vi "ma_sml_Parameter Setting for Zoom Factor.vi"(0 "zoom settings":T1={"zoom"=0, "aliasing protection"=enum."84 dB", "alias protect in transition band"=FALSE, "oversampling ratio"=1.0} {"oversampling ratio" format="%.2f"; "zoom" min=0}, 1 "Reset":bool) -> (2 "CIC Stages":i32, 3 "comb filter order":i32, 4 "interpolation":i32, 5 "filter length":i32, 6 "CFIR par":cluster{"h":dbl[], "M":i32, "N":i32} {"h" format="%.2f"}, 7 "LFIR par":cluster{"h":dbl[], "M":i32, "N":i32} {"h" format="%.2f"})   [LabVIEW 2020, in "NI_MAPro.lvlib"]
uses:
  NI_MAPro.lvlib
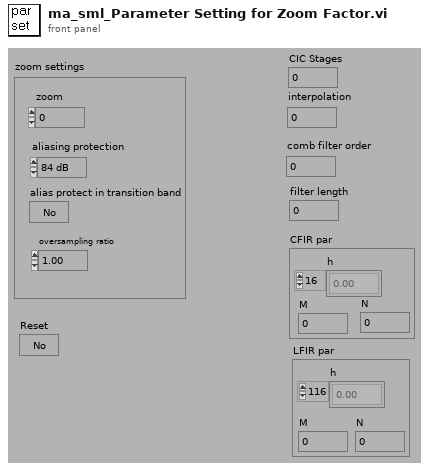
[diagram p1: front panel]
types:
  T1 = cluster{"zoom":i32, "aliasing protection":enum16{"84 dB", "96 dB", "120 dB"}, "alias protect in transition band":bool, "oversampling ratio":dbl}
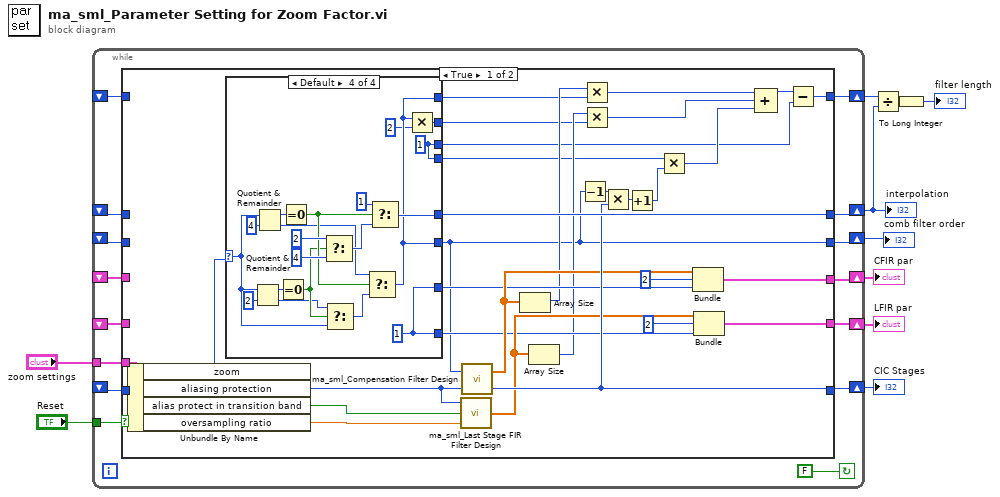
[diagram p0: block diagram]
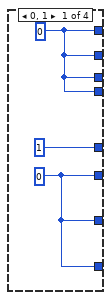
[diagram p2: hidden frame]
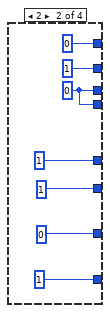
[diagram p3: hidden frame]
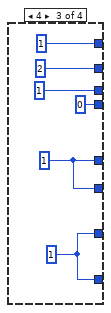
[diagram p4: hidden frame]
diagram:
  n1 = while {
    tunnel: "zoom settings" -> [w11]
    shift-left: _ -> [w14]
    shift-right: [w15] -> w4
    shift-left: _ -> [w16]
    shift-right: [w13] -> w6
    tunnel: "Reset" -> [w17]
    shift-left: _ -> [w18]
    shift-right: [w21] -> w9
    shift-left: _ -> [w19]
    shift-right: [w20] -> w3
    shift-left: _ -> [w22]
    shift-right: [w24] -> w7
    shift-left: _ -> [w23]
    shift-right: [w25] -> w8
    stop <- FALSE continue-if-true
    n2 = case shown="True" w17 {
      tunnel: [w53 w97] -> w25
      tunnel: [w52 w96] -> w24
      tunnel: w23 -> [_ w97]
      tunnel: w22 -> [_ w96]
      tunnel: [w27 w94] -> w21
      tunnel: [w50 w95] -> w20
      tunnel: w19 -> [_ w95]
      tunnel: w18 -> [_ w94]
      tunnel: [w49 w93] -> w13
      tunnel: w16 -> [_ w93]
      tunnel: [w32 w92] -> w15
      tunnel: w14 -> [_ w92]
      tunnel: w11 -> [w43 _]
      frame True {
        n3 = Unbundle By Name(w43) -> ("zoom"=w44:i32, "aliasing protection"=w51:enum16{"84 dB", "96 dB", "120 dB"}, "alias protect in transition band"=w47:bool, "oversampling ratio"=w46:dbl)
        n4 = case shown="Default" w44 {
          selector: w44 -> [_ _ _ w76]
          tunnel: [1 1 w70 w86] -> w50
          tunnel: [w58 1 w70 w74] -> w27
          tunnel: [w58 0 w71 w89] -> w42
          tunnel: [w58 1 w71 w89] -> w36
          tunnel: [w56 0 1 w74] -> w31
          tunnel: [w56 1 2 w75] -> w30
          tunnel: [w56 w59 1 w72] -> w29
          tunnel: [w56 w59 0 w72] -> w26
          frame 0, 1 {
            w56 = 0
            w58 = 0
          }
          frame 2 {
            w59 = 0
          }
          frame 4 {
            w71 = 1
            w70 = 1
          }
          frame Default {
            w72 = 1
            w89 = 1
            n5 = Quotient & Remainder(x=w76, y=2) -> (x-y*floor(x/y)=w88:i32, floor(x/y)=w77:i32)
            n6 = Quotient & Remainder(x=w76, y=4) -> (x-y*floor(x/y)=w90:i32, floor(x/y)=w78:i32)
            n7 = Equal To 0?(x=w88) -> (x = 0?=w79:bool)
            n8 = Equal To 0?(x=w90) -> (x = 0?=w81:bool)
            n9 = Select(t=2, s=w79, f=4) -> (s? t:f=w82:i32)
            n10 = Select(t=w77, s=w79, f=w76) -> (s? t:f=w80:i32)
            n11 = Select(t=w78, s=w81, f=w80) -> (s? t:f=w74:i32)
            n12 = Select(t=1, s=w81, f=w82) -> (s? t:f=w86:i32)
            n13 = Multiply(x=w74, y=2) -> (x*y=w75:i32)
          }
        }
        n14 = call "ma_sml_Last Stage FIR Filter Design.vi"("oversampling rate"=w46, "alias protect in final transition"=w47, "stop band attenuation"=w51) -> ("h"=w45:dbl[])
        n15 = call "ma_sml_Compensation Filter Design.vi"("stop band attenuation"=w51, "M"=w27) -> ("CIC stages"=w49:i32, "filter coefficients"=w48:dbl[])
        n16 = Array Size(array=w48) -> (size(s)=w34:i32)
        n17 = Array Size(array=w45) -> (size(s)=w35:i32)
        n18 = Decrement(x=w27) -> (x-1=w41:i32)
        n19 = Multiply(x=w34, y=w31) -> (x*y=w33:i32)
        n20 = Multiply(x=w35, y=w30) -> (x*y=w28:i32)
        n21 = Multiply(x=w41, y=w49) -> (x*y=w40:i32)
        n22 = Increment(x=w40) -> (x+1=w39:i32)
        n23 = Multiply(x=w26, y=w39) -> (x*y=w38:i32)
        n24 = Bundle("filter coefficients"=w48, 2, w42) -> (w53:cluster{"filter coefficients":dbl[], i32, i32})  [unwired: 1 out]
        n25 = Bundle("h"=w45, 2, w36) -> (w52:cluster{"h":dbl[], i32, i32})  [unwired: 1 out]
        n26 = Compound Arithmetic op=ADD(w33, w28, w38) -> (w37:i32)
        n27 = Subtract(x=w37, y=w29) -> (x-y=w32:i32)
      }
      frame False {
      }
    }
  }
  "interpolation" <- w3
  "comb filter order" <- w9
  "CFIR par" <- w8
  "LFIR par" <- w7
  "CIC Stages" <- w6
  n28 = Divide(x=w4, y=w3) -> (x/y=w5:dbl)
  n29 = To Long Integer(number=w5) -> (32bit integer=→"filter length":i32)
